vi "Entry.vi"(8 "error in (no error)":errorcluster, 11 "Running in":refnum<class "Running.lvclass">) -> (0 "error out":errorcluster, 3 "Running out":refnum<class "Running.lvclass">)   [LabVIEW 2013, in "Process States.lvlib" / "Running.lvclass"]
doc: "This override sends a Start Acquisition message to the Process Actor. It also sends a Log Event message to the UI, with the string \"Entering Running State\" as its payload."
uses:
  Running.lvclass
  Process State/Process State.lvclass
  <vilib>/ActorFramework/Actor/Actor.lvclass/Actor.ctl
  Process State/Process State.lvclass/Process State.ctl
  State Pattern UI/Log Event Msg/Log Event Msg.lvclass/Log Event Msg.ctl
  <vilib>/ActorFramework/Message Enqueuer/Message Enqueuer.lvclass/Message Enqueuer.ctl
  <vilib>/ActorFramework/Message Enqueuer/Enqueue.vi
  <vilib>/ActorFramework/Message Priority Queue/Priority Enqueue.vi
  State Pattern UI/Log Event Msg/Log Event Msg.lvclass
  Process Actor/Process Messages/Start Acquisition Msg/Start Acquisition Msg.lvclass
  <vilib>/ActorFramework/Actor/Actor.lvclass
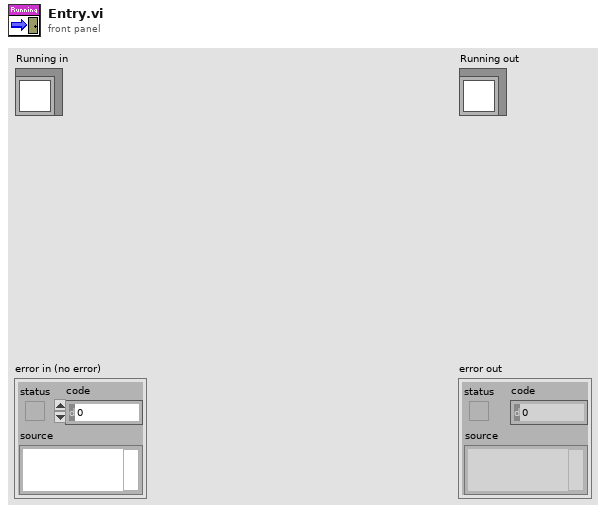
[diagram p1: front panel]
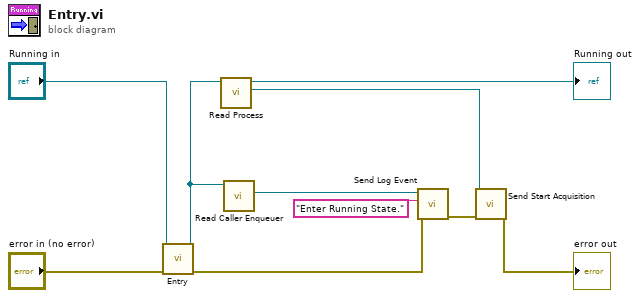
[diagram p0: block diagram]
diagram:
  n1 = call-parent "Entry.vi"("error in (no error)"="error in (no error)", "New State"="Running in") -> ("error out"=w2:errorcluster, "State out"=w5:refnum<class "Running.lvclass">)  [unwired: 8 in]
  n2 = call "Read Process.vi"("Process State in"=w5) -> ("Process Enqueuer"=w3:refnum<class "Message Enqueuer.lvclass">, "Process State out"=→"Running out":refnum<class "Running.lvclass">)  [unwired: 9 in]
  n3 = call <vilib>:"Read Caller Enqueuer.vi"("Actor"=w5) -> ("Caller Enqueuer"=w7:refnum<class "Message Enqueuer.lvclass">)  [unwired: 10 in]
  n4 = call "Send Log Event.vi"("error in (no error)"=w2, "Event Text"="Enter Running State.", "Message Enqueuer"=w7) -> ("error out"=w4:errorcluster)  [unwired: 8 in]
  n5 = call "Send Start Acquisition.vi"("error in (no error)"=w4, "Message Enqueuer"=w3) -> ("error out"=→"error out":errorcluster)  [unwired: 8 in, 1 out]
